vi "Display Actor Error.vi"(11 "error in":errorcluster) -> (4 "Shutdown":bool, 15 "error out":errorcluster)   [LabVIEW 2016, in "_Parent Actor Template.lvlib" / "_Parent Actor Template.lvclass"]
doc: "Displays any errors that are not recognized as a standard Actor error. Leaves the decision of whether to shut down Actor or attempt to continue to the user.\n\nReturns shutdown boolean TRUE for the following errors: 43, 1608, and 1556.\n\n43, 1608:\nStop on Normal Stop and Emergency Stop errors.\n\n1556:\nAlso stop if calling Actor has stopped. (invalid enqueuer error)"
uses:
  _Parent Actor Template.lvclass
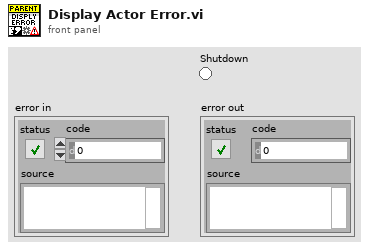
[diagram p1: front panel]
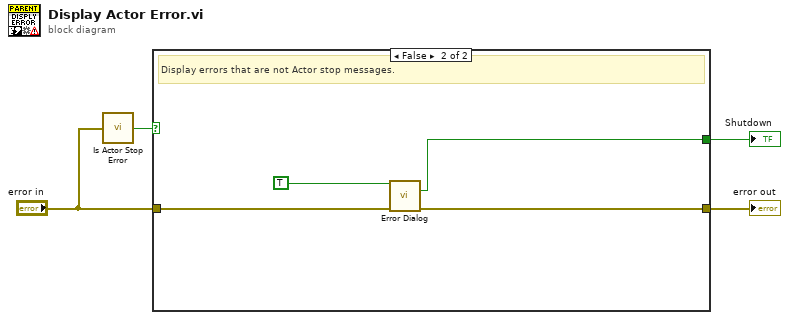
[diagram p0: block diagram]
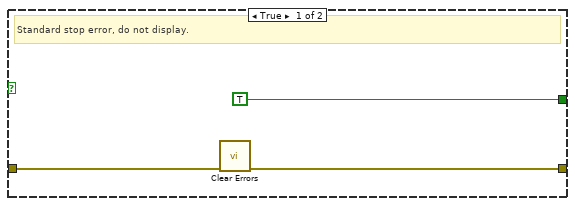
[diagram p2: hidden frame]
diagram:
  n1 = call "Is Actor Stop Error.vi"("error in"="error in") -> ("Stop Error"=w1:bool)
  n2 = case shown="False" w1 {
    tunnel: "error in" -> [w6 w9]
    tunnel: [w5 w8] -> w3
    tunnel: [TRUE ("Shutdown") w10] -> w4
    frame True {
      # "Standard stop error, do not display."
      n3 = call <vilib>:"Clear Errors.vi"("error in (no error)"=w6) -> ("error out"=w5:errorcluster)  [unwired: 5 in, 1 out]
    }
    frame False {
      # "Display errors that are not Actor stop messages."
      n4 = call "Error Dialog.vi"("Clear Error?"=TRUE, "error in"=w9) -> ("Shutdown"=w10:bool, "error out"=w8:errorcluster)  [unwired: 12 in]
    }
  }
  "Shutdown" <- w4
  "error out" <- w3
